vi "UMLEditor createWizardScriptFile_UpdateList.vi"(8 "error in (no error)":errorcluster, 9 "UpdateLastLine(False)":bool, 10 "String":string, 11 "Progress":refnum<vi>) -> (0 "error out":errorcluster)   [LabVIEW 2020]
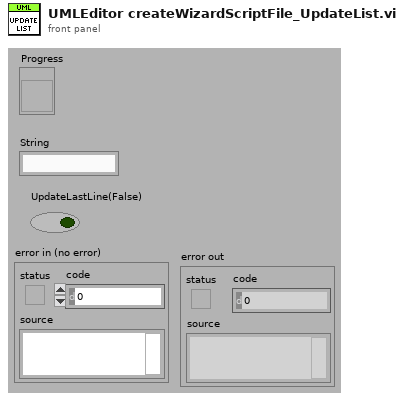
[diagram p1: front panel]
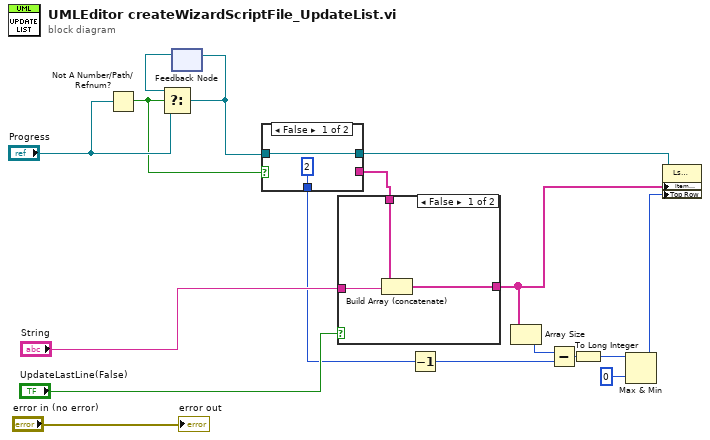
[diagram p0: block diagram]
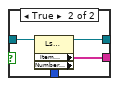
[diagram p2: hidden frame]
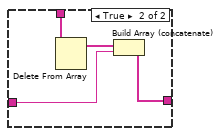
[diagram p3: hidden frame]
diagram:
  n1 = Not A Number/Path/Refnum?(number/path/refnum="Progress") -> (NaN/Path/Refnum?=w3:bool)
  n2 = feedback #1() -> (w7:refnum<vi>)  [unwired: 1 in]
  n3 = Select(t=w7, s=w3, f="Progress") -> (s? t:f=w6:refnum<vi>)
  n4 = feedback-in #1(w6) -> ()
  n5 = case shown="False" w3 {
    tunnel: [w19 w23] -> w16
    tunnel: [u32 2 ("Number of Rows") w22] -> w2
    tunnel: [_ w21] -> w9
    tunnel: w6 -> [w19 w20]
    frame False {
    }
    frame True {
      n6 = property on="Property Node" class="LstBox (strict)"(reference=w20) -> (reference out=w23:refnum<vi>, "Item Names"=w21:string[], "Number of Rows"=w22:u32)  [unwired: 1 in, 1 out]
    }
  }
  n7 = case shown="False" "UpdateLastLine(False)" {
    tunnel: "String" -> [w26 w28]
    tunnel: [w25 w27] -> w14
    tunnel: w9 -> [w24 w30]
    frame False {
      n8 = Build Array (concatenate)(w24, w26) -> (w25:string[])
    }
    frame True {
      n9 = Delete From Array(array=w30) -> (array with subset deleted=w29:string[])  [unwired: 2 in, 1 out]
      n10 = Build Array (concatenate)(w29, w28) -> (w27:string[])
    }
  }
  n11 = Decrement(x=w2) -> (x-1=w1:u32)
  n12 = Array Size(array=w14) -> (size(s)=w10:i32)
  n13 = Subtract(x=w10, y=w1) -> (x-y=w11:u32)
  n14 = To Long Integer(number=w11) -> (32bit integer=w13:i32)
  n15 = Max & Min(x=w13, y=0) -> (max(x,y)=w15:i32)  [unwired: 1 out]
  n16 = property on="Property Node" class="LstBox (strict)"(reference=w16, "Item Names"=w14, "Top Row"=w15) -> ()  [unwired: 1 in, 2 out]
  "error out" <- "error in (no error)"
